vi "Write Size.vi"(8 "error in (no error)":errorcluster, 10 "Size":i64, 11 "file in":refnum<class "node.lvclass">) -> (0 "error out":errorcluster, 3 "file out":refnum<class "node.lvclass">)   [LabVIEW 2023, in "d7.lvlib" / "node.lvclass"]
uses:
  node.lvclass
  node.lvclass/node.ctl
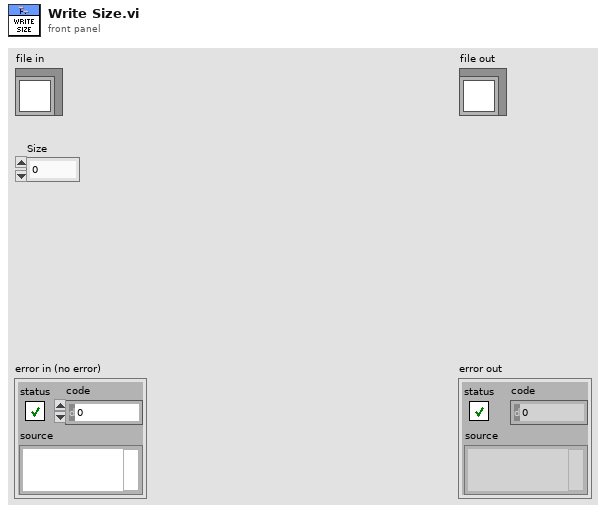
[diagram p1: front panel]
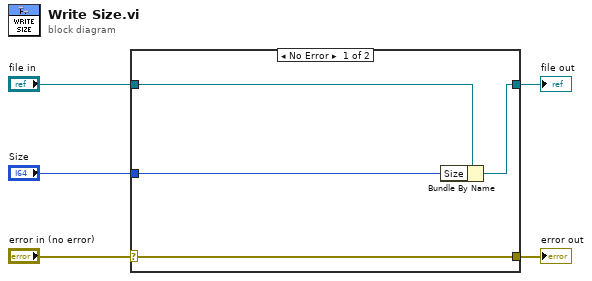
[diagram p0: block diagram]
diagram:
  n1 = case shown="No Error" "error in (no error)" {
    selector: "error in (no error)" -> [w9 w10]
    tunnel: [w9 w10] -> w4
    tunnel: [w7 w11] -> w2
    tunnel: "file in" -> [w8 w11]
    tunnel: "Size" -> [w6 _]
    frame No Error {
      n2 = Bundle By Name(cluster=w8, "Size"=w6) -> (w7:refnum<class "node.lvclass">)
    }
    frame Error {
    }
  }
  "error out" <- w4
  "file out" <- w2
